vi "SIMPLE_Read_Stat.vi"() -> ()   [LabVIEW 2016]
uses:
  <vilib>/Instr/_visa.llb/VISA Set IO Buffer Mask.ctl
  <vilib>/Utility/miscctls.llb/LVPointTypeDef.ctl
  <vilib>/Instr/_visa.llb/VISA Configure Serial Port (Instr).vi
  GEN_2.lvlib
  GEN2_Stat_Addr.ctl
panel:
  in  "Address":T1[](array[typedef])=[9, 10, 11, 12, 13] items=["Torque Enable", "Homing Complete", "Goal Id", "Goal Iq", "Goal Velo", "Goal Posi", "Present Id", "Present Iq", "Present Velo", "Present Posi", "Bus Voltage", "Temperature Winding", "Temperature MOSFET", "Temperature IC", "Error Status", "Iq_Temps"]
  out "ERROR":u8
  out "value":dbl[](array[numeric])=[2903.94775390625, 24.112640380859375, 25.25, 24.875, 27.875]
  in  "ID":u8=1 format="%x"
  in  "write":bool
  in  "Baud rate":u32=8000000
  in  "Com port":refnum<visa-resource-name>="COM8"
  in  "stop":bool
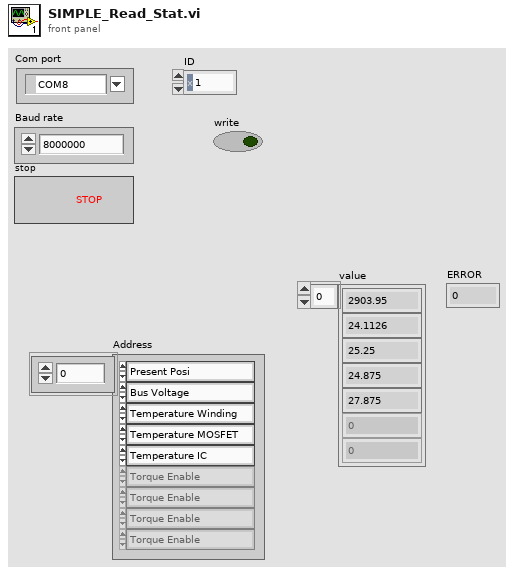
[diagram p1: front panel]
types:
  T1 = typedef "GEN_2.lvlib/GEN2_Stat_Addr.ctl" = u8
  T2 = typedef "LVPointTypeDef.ctl" = cluster{"Horizontal":i16, "Vertical":i16}
  T3 = typedef "VISA Set IO Buffer Mask.ctl" = u16
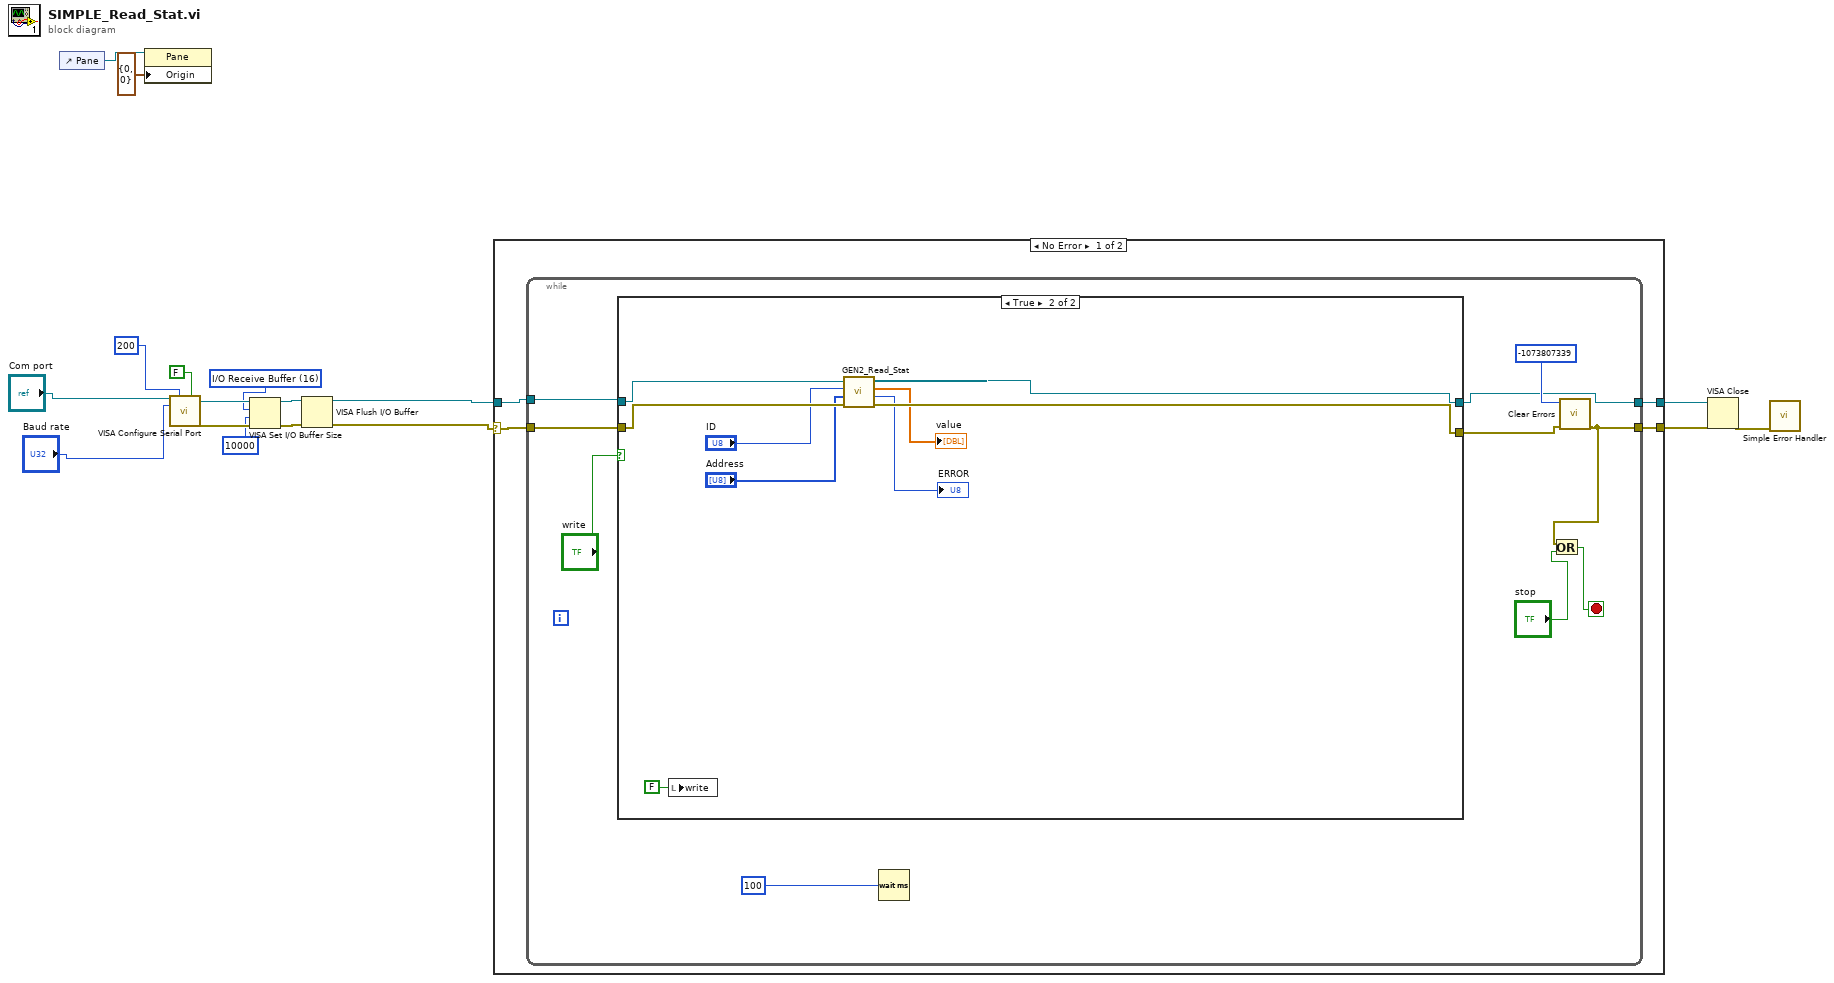
[diagram p0: block diagram]
diagram:
  w9 = T3 16 items=["I/O Receive Buffer"=16, "I/O Transmit Buffer"=32, "I/O Receive and Transmit Buffer"=48] ("Mask")
  n1 = control-ref of="Pane"() -> (w4:refnum<vi>)
  n2 = property class="Pane"(reference=w4, "Origin"=T2 {"Horizontal"=0, "Vertical"=0}) -> ()  [unwired: 1 in, 2 out]
  n3 = call-poly "VISA Configure Serial Port"("VISA resource name"="Com port", "timeout (10sec)"=u32 200, "Enable Termination\nChar (T)"=FALSE ("Enable Termination\nChar (T)"), "baud rate (9600)"="Baud rate") -> ("VISA resource name out"=w10:refnum<visa-resource-name>, "error out"=w13:errorcluster)  [unwired: 10 in]
  n4 = VISA Set I/O Buffer Size(VISA resource name=w10, mask (16)=w9, size (4096)=u32 10000, error in (no error)=w13) -> (VISA resource name out=w11:refnum<visa-resource-name>, error out=w12:errorcluster)
  n5 = VISA Flush I/O Buffer(VISA resource name=w11, error in (no error)=w12) -> (VISA resource name out=w1:refnum<visa-resource-name>, error out=w2:errorcluster)  [unwired: 1 in]
  n6 = case shown="No Error" w2 {
    selector: w2 -> [w18 w43]
    tunnel: [w21 w43] -> w17
    tunnel: w1 -> [w20 w44]
    tunnel: [w19 w44] -> w15
    frame No Error {
      n7 = while {
        tunnel: w20 -> [w27]
        tunnel: w18 -> [w26]
        tunnel: [w24] -> w19
        tunnel: [w25] -> w21
        stop <- w30 stop-if-true
        n8 = case shown="True" "write" {
          tunnel: w26 -> [w33 w42]
          tunnel: w27 -> [w32 w41]
          tunnel: [w32 w38] -> w24
          tunnel: [w33 w39] -> w23
          frame False {
          }
          frame True {
            n9 = local write "write"(FALSE ("write")) -> ()
            n10 = call "GEN2_Read_Stat.vi"("error in (no error)"=w42, "Stat Address"="Address", "ID"="ID", "VISA Refnum in"=w41) -> ("error out"=w39:errorcluster, "ERROR"=→"ERROR":u8, "Data"=→"value":dbl[], "VISA Refnum out"=w38:refnum<visa-resource-name>)  [unwired: 4 in]
          }
        }
        n11 = Wait (ms)(milliseconds to wait=u32 100) -> ()  [unwired: 1 out]
        n12 = call <vilib>:"Clear Errors.vi"("error in (no error)"=w23, "specific error code to clear (0: all)"=-1073807339) -> ("error out"=w25:errorcluster)  [unwired: 4 in, 1 out]
        n13 = Or(x=w25, y="stop") -> (x .or. y?=w30:bool)
      }
    }
    frame Error {
    }
  }
  n14 = VISA Close(VISA resource name=w15, error in (no error)=w17) -> (error out=w7:errorcluster)
  n15 = call <vilib>:"Simple Error Handler.vi"("error in (no error)"=w7) -> ()  [unwired: 4 in, 5 out]
